vi "Actor Core.vi"(8 "error in":errorcluster, 11 "IEventAggregator in":refnum<class "IEventAggregator.lvclass">) -> (0 "error out":errorcluster, 3 "Actor out":refnum<class "Actor.lvclass">)   [LabVIEW 2015, in "ActorEvents.lvlib" / "IEventAggregator.lvclass"]
doc: "(<B>Filename</B>: Actor Framework.lvlib:Actor.lvclass:Actor Core.vi)\n\nReceives messages to the actor, reacts to them, and initiates any error handling that may shut the actor down.\n\nDescendant classes may override this VI to append parallel tasks for the actor to complete while it handles messages. Overrides use the Call Parent Method node."
uses:
  IEventAggregator.lvclass
  <vilib>/ActorFramework/Actor/Actor.lvclass
  IEventAggregator.lvclass/IEventAggregator.ctl
  <vilib>/ActorFramework/Actor/Actor.lvclass/Actor.ctl
  <vilib>/ActorFramework/Message Enqueuer/Message Enqueuer.lvclass/Message Enqueuer.ctl
  <vilib>/ActorFramework/Message Enqueuer/Init from Existing Queue.vi
  <vilib>/ActorFramework/Message Enqueuer/Enqueue.vi
  <vilib>/ActorFramework/Message Priority Queue/Priority Enqueue.vi
  IObserver/IObserver/IObserver.lvclass
  <vilib>/ActorFramework/Message Enqueuer/Message Enqueuer.lvclass
  AutoEventActor Messages/Launch Event Handlers Msg/Launch Event Handlers Msg.lvclass
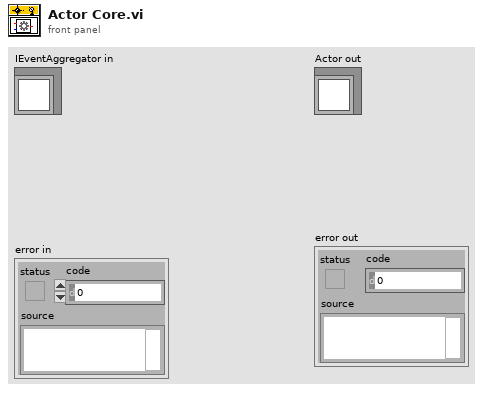
[diagram p1: front panel]
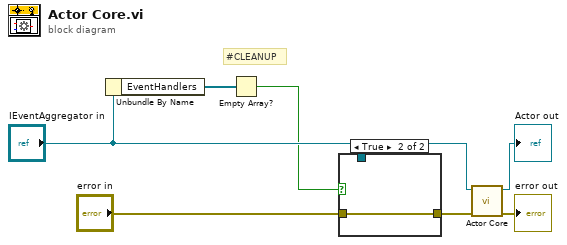
[diagram p0: block diagram]
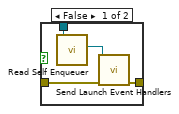
[diagram p2: hidden frame]
diagram:
  # "#CLEANUP"
  n1 = Unbundle By Name("IEventAggregator in") -> ("EventHandlers"=w4:refnum<class "IEventHandler.lvclass">[])
  n2 = Empty Array?(array=w4) -> (empty?=w1:bool)
  n3 = case shown="True" w1 {
    tunnel: "error in" -> [w11 w12]
    tunnel: [w10 w12] -> w3
    tunnel: "IEventAggregator in" -> [w9 _]
    frame False {
      n4 = call <vilib>:"Read Self Enqueuer.vi"("Actor"=w9) -> ("Self Enqueuer"=w8:refnum<class "Message Enqueuer.lvclass">)  [unwired: 10 in]
      n5 = call "Send Launch Event Handlers.vi"("error in (no error)"=w11, "Message Enqueuer (EventAggregator)"=w8) -> ("error out"=w10:errorcluster)  [unwired: 8 in, 1 out]
    }
    frame True {
    }
  }
  n6 = call-parent "Actor Core.vi"("error in"=w3, "Actor in"="IEventAggregator in") -> ("error out"=→"error out":errorcluster, "Actor out"=→"Actor out":refnum<class "Actor.lvclass">)  [unwired: 8 in]
